vi "Piezo Message Loop.vi"(8 "error in (no error)":errorcluster, 10 "Data Notifiers":T1, 11 "Message Queues":T2) -> (0 "error out":errorcluster)   [LabVIEW 2013, in "Piezo.lvlib"]
uses:
  Piezo.lvlib
  support/Message Queue/All Message Queues.ctl
  support/Message Queue/Message Cluster.ctl
  support/Data Notifiers/All Data Notifiers.ctl
  Acquisition/APD Notifier Cluster.ctl
  Piezo display.ctl
  XY/XY Display.ctl
  Capacitive/Capacitive Signal Cluster.ctl
  Feedback/Error Signal.ctl
  Piezo State.ctl
  piezo new/Hardware Configuration Piezo.ctl
  support/Message Queue/Enqueue Message (Single).vi
  <vilib>/Utility/error.llb/Error Cluster From Error Code.vi
  <vilib>/ErrorRing/Error Ring.xnode
  support/Message Queue/Message Queue.lvlib
  Acquisition/Acquisition.lvlib
  XY/XY.lvlib
  support/Data Notifiers/Data Notifiers.lvlib
  Capacitive/Capacitive.lvlib
  Feedback/Feedback.lvlib
panel:
  out "ACTUAL POSITION \n[MICRON]":dbl[](array[numeric])
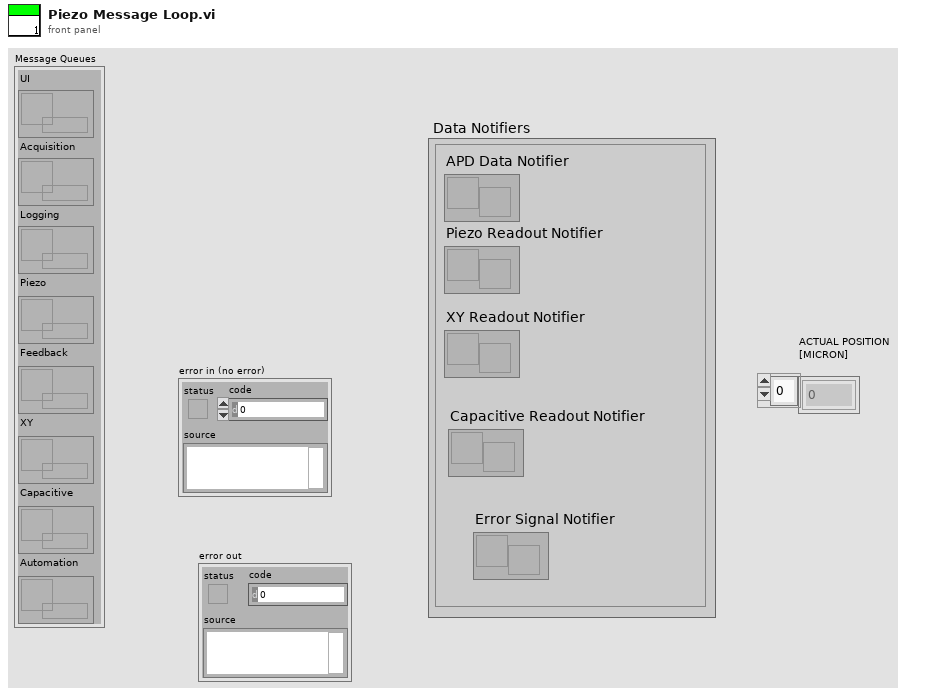
[diagram p1: front panel]
types:
  T1 = typedef "Data Notifiers.lvlib/All Data Notifiers.ctl" = cluster{"APD Data Notifier":refnum<notifier>, "Piezo Readout Notifier":refnum<notifier>, "XY Readout Notifier":refnum<notifier>, "Capacitive Readout Notifier":refnum<notifier>, "Error Signal Notifier":refnum<notifier>}
  T2 = typedef "Message Queue.lvlib/All Message Queues.ctl" = cluster{"UI":refnum<queue>, "Acquisition":refnum<queue>, "Logging":refnum<queue>, "Piezo":refnum<queue>, "Feedback":refnum<queue>, "XY":refnum<queue>, "Capacitive":refnum<queue>, "Automation":refnum<queue>}
  T3 = typedef "Piezo.lvlib/Hardware Configuration Piezo.ctl" = cluster{"DAQmx Channel":tag, "Max Input":dbl, "Min Input":dbl, "Samples per ch.":dbl, "Setpoint (um)":dbl, "DAQmx Task":refnum<k21>}
  T4 = typedef "Piezo.lvlib/Piezo State.ctl" = enum16{"Idle", "Acquiring"}
  T5 = typedef "Acquisition.lvlib/APD Notifier Cluster.ctl" = cluster{"data":dbl[][], "t0":i32}
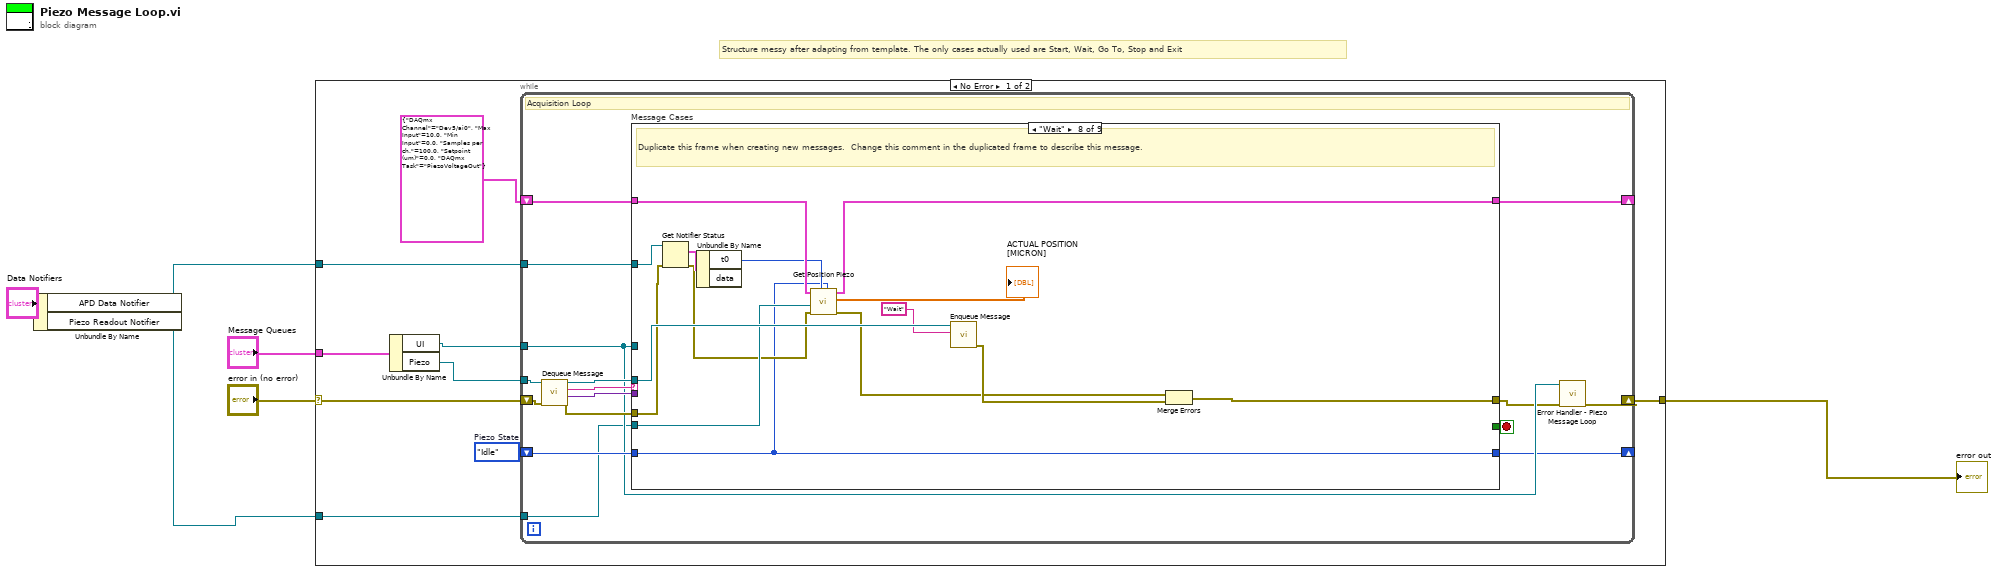
[diagram p0: block diagram]
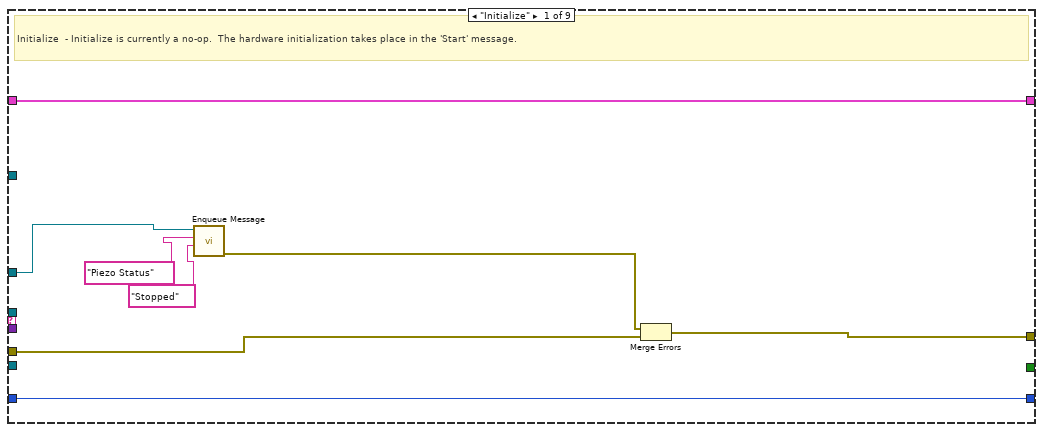
[diagram p2: hidden frame]
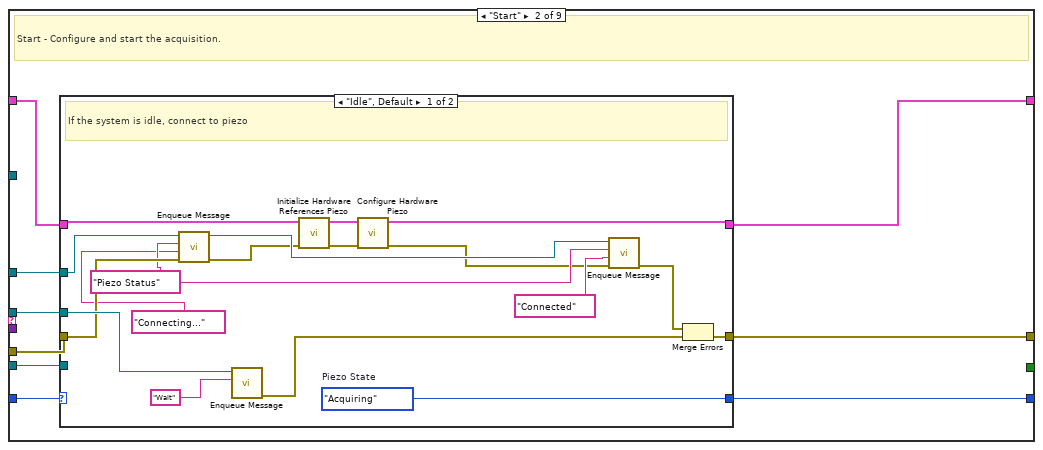
[diagram p3: hidden frame]
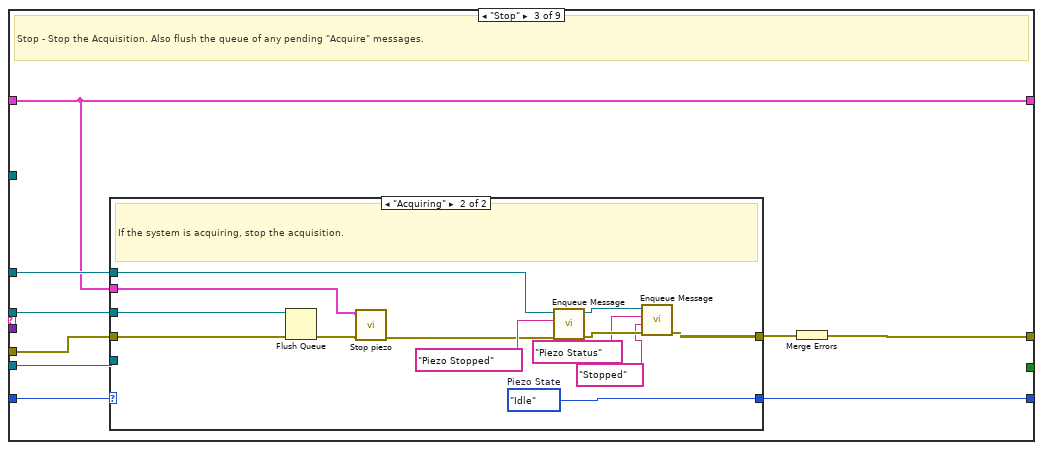
[diagram p5: hidden frame]
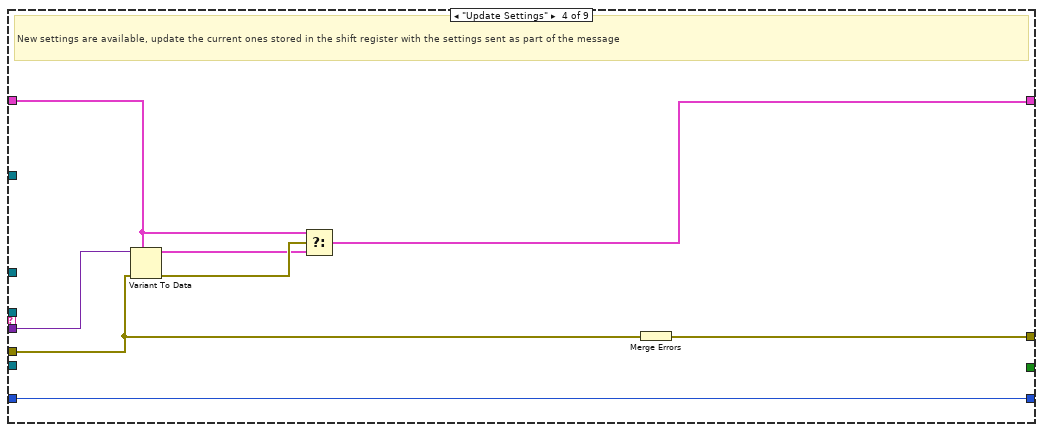
[diagram p7: hidden frame]
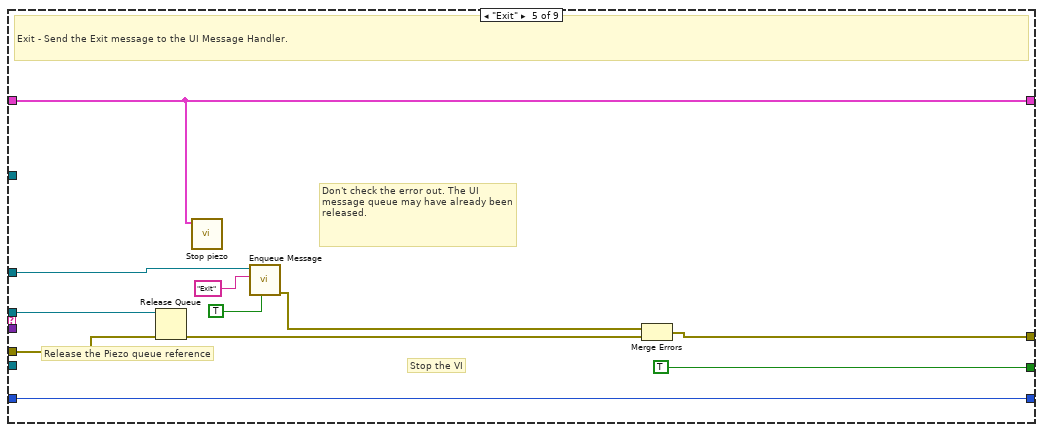
[diagram p8: hidden frame]
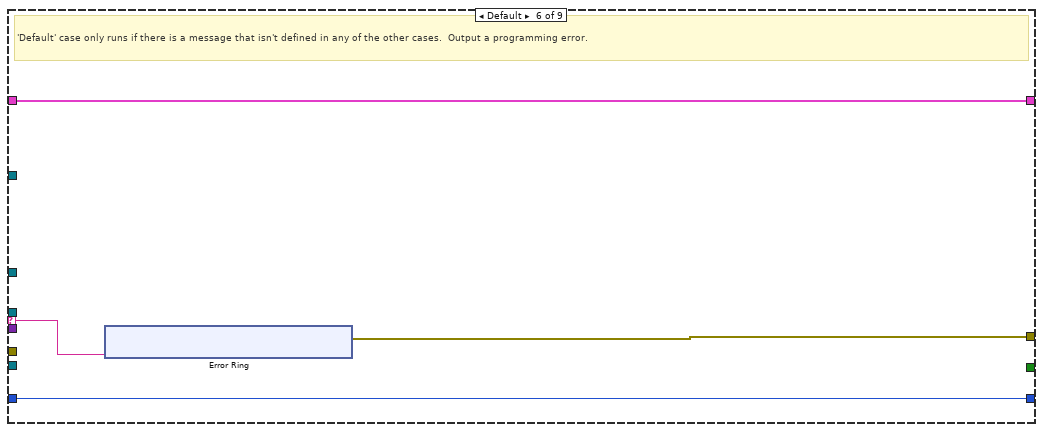
[diagram p9: hidden frame]
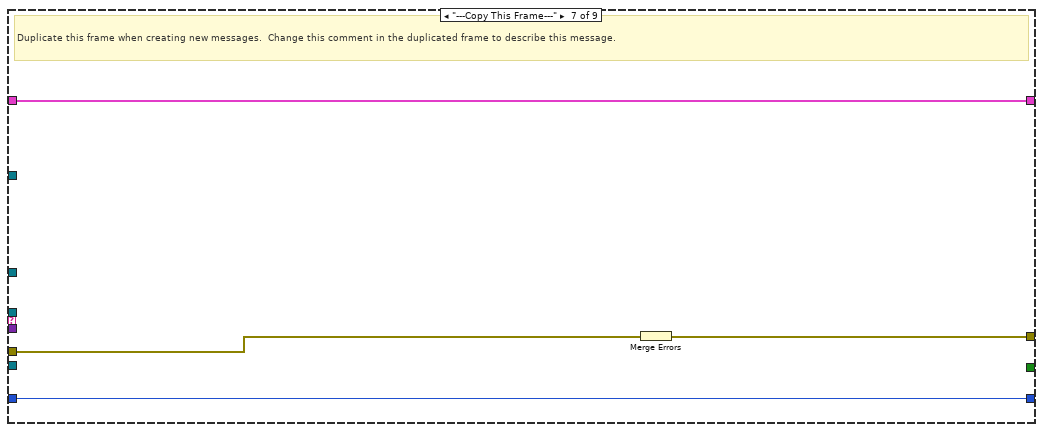
[diagram p10: hidden frame]
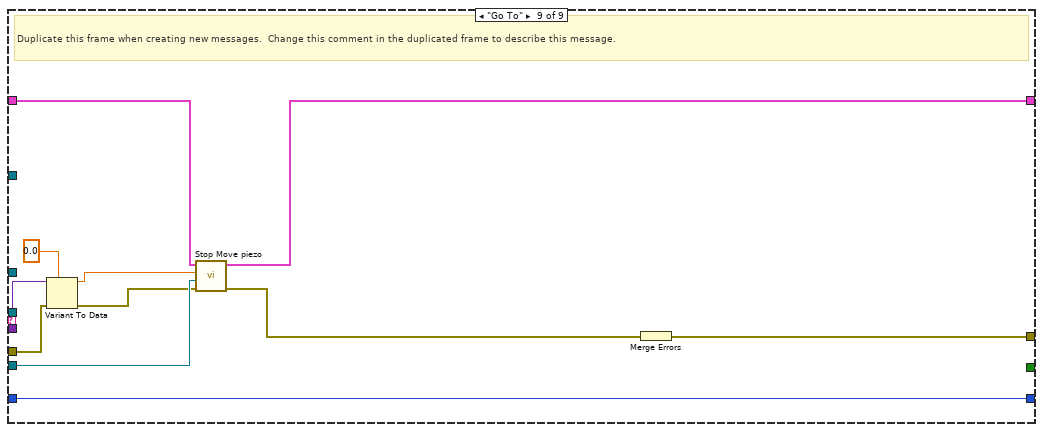
[diagram p11: hidden frame]
diagram:
  # "Structure messy after adapting from template. The only cases actually used are Start, Wait, Go To, Stop and Exit"
  n1 = Unbundle By Name("Data Notifiers") -> ("APD Data Notifier"=w2:refnum<notifier>, "Piezo Readout Notifier"=w1:refnum<notifier>)
  n2 = case shown="No Error" "error in (no error)" {
    selector: "error in (no error)" -> [w10 w154]
    tunnel: "Message Queues" -> [w15 _]
    tunnel: [w13 w154] -> w5
    tunnel: w1 -> [w9 _]
    tunnel: w2 -> [w8 _]
    frame No Error {
      w11 = Piezo_State."Idle"  # Piezo State
      n3 = Unbundle By Name(w15) -> ("UI"=w12:refnum<queue>, "Piezo"=w14:refnum<queue>)
      n4 = while {
        tunnel: w14 -> [w24]
        shift-right: [w19] -> _
        shift-left: T3 {"DAQmx Channel"="Dev5/ai0", "Max Input"=10.0, "Min Input"=0.0, "Samples per ch."=100.0, "Setpoint (um)"=0.0, "DAQmx Task"="PiezoVoltageOut"} ("Hardware Configuration") -> [w31]
        shift-right: [w21] -> w13
        shift-left: w10 -> [w29]
        tunnel: w12 -> [w22]
        shift-right: [w20] -> _
        shift-left: w11 -> [w23]
        tunnel: w9 -> [w17]
        tunnel: w8 -> [w16]
        stop <- w30 stop-if-true
        # "Acquisition Loop"
        n5 = call "Dequeue Message.vi"("error in (no error)"=w29, "Message Queue"=w24) -> ("error out"=w28:errorcluster, "Message Data"=w26:variant, "Message"=w27:string, "dup Message Queue"=w25:refnum<queue>)  [unwired: 6 in]
        n6 = case "Message Cases" shown="\"Wait\"" w27 {
          selector: w27 -> [_ _ _ _ _ w116 _ _ _]
          tunnel: w25 -> [_ w45 w76 _ w108 _ _ w141 _]
          tunnel: w28 -> [w38 w46 w77 w96 w110 _ w127 w138 w149]
          tunnel: [w39 w48 w78 w101 w111 w115 w126 w142 w153] -> w18
          tunnel: w31 -> [w36 w47 w71 w97 w102 w113 w124 w135 w148]
          tunnel: [_ _ _ _ TRUE _ _ _ _] -> w30
          tunnel: w26 -> [_ _ _ w100 _ _ _ _ w151]
          tunnel: w22 -> [w34 w41 w75 _ w104 _ _ _ _]
          tunnel: w23 -> [w37 w44 w74 w95 w107 w114 w125 w130 w152]
          tunnel: [w37 w43 w73 w95 w107 w114 w125 w130 w152] -> w20
          tunnel: [w36 w42 w71 w94 w102 w113 w124 w134 w147] -> w19
          tunnel: w17 -> [_ w40 w70 _ _ _ _ w133 w145]
          tunnel: w16 -> [_ _ _ _ _ _ _ w137 _]
          frame "Initialize" {
            # "Initialize  - Initialize is currently a no-op.  The hardware initialization takes place in the 'Start' message."
            n7 = call-poly "Enqueue Message.vi"("Message Data"="Stopped" ("Message"), "Message"="Piezo Status", "Message Queue"=w34) -> ("error out"=w33:errorcluster)  [unwired: 7 in, 1 out]
            n8 = Merge Errors(w33, w38) -> (w39:errorcluster)
          }
          frame "Start" {
            # "Start - Configure and start the acquisition."
            n9 = case shown="\"Idle\", Default" w44 {
              selector: w44 -> [_ w67]
              tunnel: [w66 w69] -> w48
              tunnel: w47 -> [w52 w68]
              tunnel: w46 -> [w58 w69]
              tunnel: w45 -> [w63 _]
              tunnel: [w50 w68] -> w42
              tunnel: [w65 w67] -> w43
              tunnel: w41 -> [w59 _]
              tunnel: w40 -> [_ _]
              frame "Idle", Default {
                w56 = "Piezo Status" ("Message")
                w65 = Piezo_State."Acquiring"  # Piezo State
                # "If the system is idle, connect to piezo"
                n10 = call-poly "Enqueue Message.vi"("error in (no error)"=w58, "Message Data"="Connecting..." ("Message"), "Message"=w56, "Message Queue"=w59) -> ("error out"=w51:errorcluster, "dup Message Queue"=w57:refnum<queue>)  [unwired: 6 in]
                n11 = call-poly "Enqueue Message.vi"("Message"="Wait", "Message Queue"=w63) -> ("error out"=w62:errorcluster)  [unwired: 8 in, 1 out]
                n12 = call "Initialize Hardware References Piezo.vi"("error in (no error)"=w51, "Hardware Configuration"=w52) -> ("error out"=w54:errorcluster, "Hardware Configuration 2"=w53:T3)  [unwired: 8 in]
                n13 = call "Configure Hardware Piezo.vi"("error in (no error)"=w54, "Hardware Configuration in"=w53) -> ("error out"=w49:errorcluster, "Hardware Configuration out"=w50:T3)  [unwired: 8 in]
                n14 = call-poly "Enqueue Message.vi"("error in (no error)"=w49, "Message Data"="Connected" ("Message"), "Message"=w56, "Message Queue"=w57) -> ("error out"=w61:errorcluster)  [unwired: 6 in, 1 out]
                n15 = Merge Errors(w61, w62) -> (w66:errorcluster)
              }
              frame "Acquiring" {
                # "The system is already acquiring. Ignore the \"Start\" message."
              }
            }
          }
          frame "Stop" {
            # "Stop - Stop the Acquisition. Also flush the queue of any pending \"Acquire\" messages."
            n16 = case shown="\"Acquiring\"" w74 {
              selector: w74 -> [w80 _]
              tunnel: w77 -> [w79 w81]
              tunnel: w71 -> [_ w82]
              tunnel: w76 -> [_ w93]
              tunnel: w75 -> [_ w92]
              tunnel: [w80 w90] -> w73
              tunnel: [w79 w87] -> w72
              tunnel: w70 -> [_ _]
              frame "Idle", Default {
                # "The system is already idle. Ignore the \"Stop\" message."
              }
              frame "Acquiring" {
                w90 = Piezo_State."Idle"  # Piezo State
                # "If the system is acquiring, stop the acquisition."
                n17 = Flush Queue(queue=w93, error in (no error)=w81) -> (error out=w84:errorcluster)  [unwired: 2 out]
                n18 = call "Stop piezo.vi"("error in (no error)"=w84, "Hardware Configuration"=w82) -> ("error out"=w83:errorcluster)  [unwired: 9 in]
                n19 = call-poly "Enqueue Message.vi"("error in (no error)"=w83, "Message"="Piezo Stopped", "Message Queue"=w92) -> ("error out"=w88:errorcluster, "dup Message Queue"=w89:refnum<queue>)  [unwired: 7 in]
                n20 = call-poly "Enqueue Message.vi"("error in (no error)"=w88, "Message Data"="Stopped" ("Message"), "Message"="Piezo Status", "Message Queue"=w89) -> ("error out"=w87:errorcluster)  [unwired: 6 in, 1 out]
              }
            }
            n21 = Merge Errors(w72) -> (w78:errorcluster)
          }
          frame "Update Settings" {
            # "New settings are available, update the current ones stored in the shift register with the settings sent as part of the message"
            n22 = Variant To Data(error in=w96, type=w97, Variant=w100) -> (data=w98:T3, error out=w99:errorcluster)
            n23 = Select(t=w97, s=w99, f=w98) -> (s? t:f=w94:T3)
            n24 = Merge Errors(w96) -> (w101:errorcluster)
          }
          frame "Exit" {
            # "Don't check the error out. The UI message queue may have already been released."
            # "Release the Piezo queue reference"
            # "Stop the VI"
            # "Exit - Send the Exit message to the UI Message Handler."
            n25 = Release Queue(queue=w108, error in (no error)=w110) -> (error out=w109:errorcluster)  [unwired: 1 in, 2 out]
            n26 = call "Stop piezo.vi"("Hardware Configuration"=w102) -> ()  [unwired: 10 in, 1 out]
            n27 = call-poly "Enqueue Message.vi"("Priority Message? (F)"=TRUE, "Message"="Exit", "Message Queue"=w104) -> ("error out"=w103:errorcluster)  [unwired: 7 in, 1 out]
            n28 = Merge Errors(w103, w109) -> (w111:errorcluster)
          }
          frame Default {
            # "'Default' case only runs if there is a message that isn't defined in any of the other cases.  Output a programming error."
            n29 = xnode "Error Ring"("parameter 0"=w116) -> ("error out"=w115:errorcluster)
          }
          frame "---Copy This Frame---" {
            # "Duplicate this frame when creating new messages.  Change this comment in the duplicated frame to describe this message."
            n30 = Merge Errors(w127) -> (w126:errorcluster)
          }
          frame "Wait" {
            # "Duplicate this frame when creating new messages.  Change this comment in the duplicated frame to describe this message."
            n31 = Get Notifier Status(notifier=w137, error in (no error)=w138) -> (current notification=w136:T5, error out=w132:errorcluster)  [unwired: 3 out]
            n32 = Unbundle By Name(w136) -> ("t0"=w131:i32)  [unwired: 1 out]
            n33 = call "Get Position Piezo.vi"("Piezo State"=w130, "Counter Time"=w131, "error in (no error)"=w132, "notifier out"=w133, "Hardware Configuration"=w135) -> ("error out"=w129:errorcluster, "ACTUAL POSITION \n[MICRON]"=→"ACTUAL POSITION \n[MICRON]":dbl[], "Hardware Configuration 2"=w134:T3)  [unwired: 2 in, 2 out]
            n34 = call-poly "Enqueue Message.vi"("Message"="Wait", "Message Queue"=w141) -> ("error out"=w139:errorcluster)  [unwired: 8 in, 1 out]
            n35 = Merge Errors(w129, w139) -> (w142:errorcluster)
          }
          frame "Go To" {
            # "Duplicate this frame when creating new messages.  Change this comment in the duplicated frame to describe this message."
            n36 = Variant To Data(error in=w149, type=sgl 0.0, Variant=w151) -> (data=w146:sgl, error out=w144:errorcluster)
            n37 = call "Stop Move piezo.vi"("error in (no error)"=w144, "notifier out"=w145, "MOVE TO [MICRON]"=w146, "Hardware Configuration in"=w148) -> ("error out"=w143:errorcluster, "Hardware Configuration out"=w147:T3)  [unwired: 6 in]
            n38 = Merge Errors(w143) -> (w153:errorcluster)
          }
        }
        n39 = call "Error Handler - Piezo Message Loop.vi"("error in (no error)"=w18, "Message Queue"=w22) -> ("dup error in"=w21:errorcluster)  [unwired: 8 in, 1 out]
      }
    }
    frame Error {
    }
  }
  "error out" <- w5
